vi "Parse Message Buffer.vi"(7 "flush buffer":bool, 8 "error in":errorcluster, 11 "string in":string) -> (0 "error out":errorcluster, 1 "valid":bool, 3 "message":T1)   [LabVIEW 2017, in "Lock-In Amplifier Example Shared.lvlib"]
uses:
  Lock-In Amplifier Example Shared.lvlib
  message.ctl
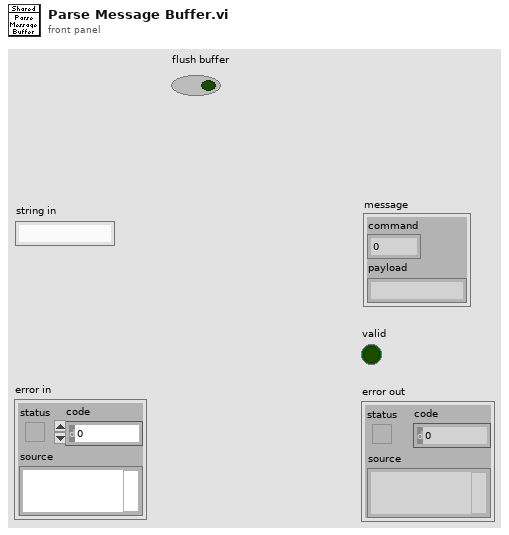
[diagram p1: front panel]
types:
  T1 = typedef "Lock-In Amplifier Example Shared.lvlib/message.ctl" = cluster{"command":u32, "payload":string}
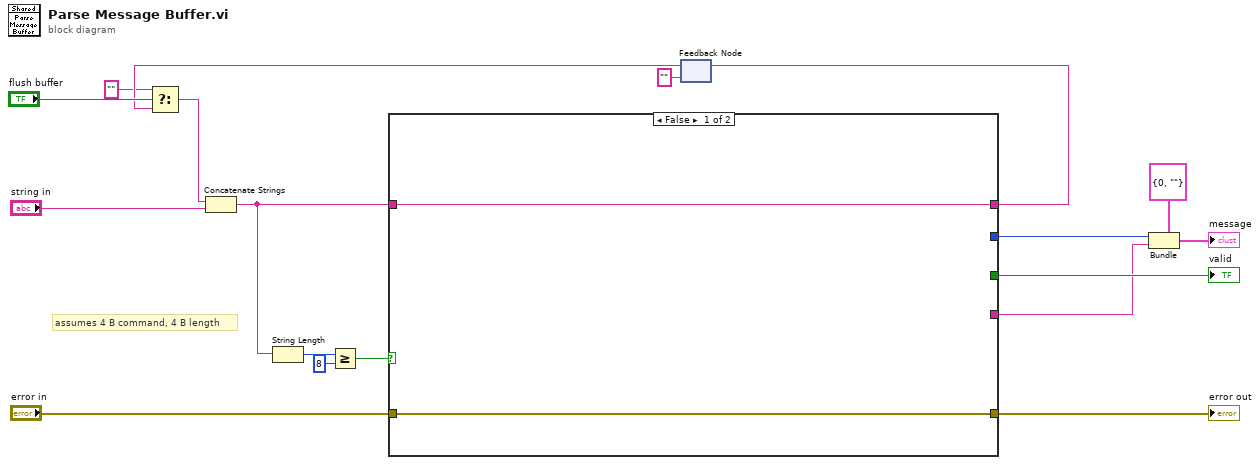
[diagram p0: block diagram]
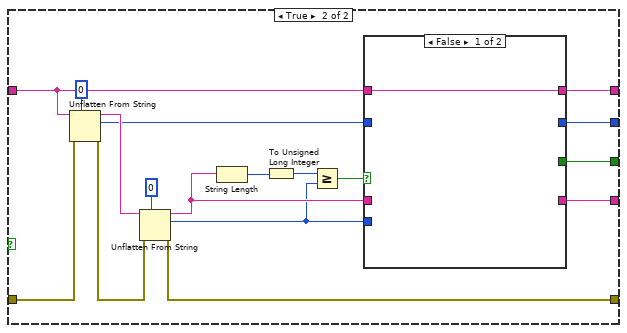
[diagram p2: hidden frame]
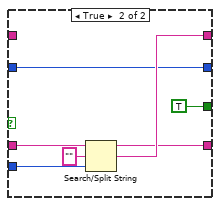
[diagram p3: hidden frame]
diagram:
  # "assumes 4 B command, 4 B length"
  n1 = feedback #1("") -> (w4:string)
  n2 = Select(t="", s="flush buffer", f=w4) -> (s? t:f=w2:string)
  n3 = Concatenate Strings(w2, "string in") -> (w13:string)
  n4 = String Length(string=w13) -> (length=w15:i32)
  n5 = Greater Or Equal?(x=w15, y=8) -> (x >= y?=w17:bool)
  n6 = case shown="False" w17 {
    tunnel: w13 -> [w20 w31]
    tunnel: [_ w30] -> w14
    tunnel: "error in" -> [w19 w29]
    tunnel: [w19 w27] -> w11
    tunnel: [w20 w24] -> w6
    tunnel: [_ w23] -> w9
    tunnel: [_ w21] -> w10
    frame False {
    }
    frame True {
      n7 = Unflatten From String(type=u32 0 ("offset (0)"), binary string=w31, error in (no error)=w29) -> (rest of the binary string=w36:string, value=w22:u32, error out=w28:errorcluster)  [unwired: 2 in]
      n8 = Unflatten From String(type=u32 0 ("offset (0)"), binary string=w36, error in (no error)=w28) -> (rest of the binary string=w26:string, value=w25:u32, error out=w27:errorcluster)  [unwired: 2 in]
      n9 = String Length(string=w26) -> (length=w34:i32)
      n10 = To Unsigned Long Integer(number=w34) -> (unsigned 32bit integer=w33:u32)
      n11 = Greater Or Equal?(x=w33, y=w25) -> (x >= y?=w32:bool)
      n12 = case shown="False" w32 {
        tunnel: w31 -> [w38 _]
        tunnel: [w38 w42] -> w24
        tunnel: [_ TRUE] -> w30
        tunnel: w26 -> [_ w45]
        tunnel: w25 -> [_ w44]
        tunnel: [_ w41] -> w23
        tunnel: w22 -> [_ w39]
        tunnel: [_ w39] -> w21
        frame False {
        }
        frame True {
          n13 = Search/Split String(string=w45, search string/char (-)="", offset (0)=w44) -> (substring before match=w41:string, match + rest of string=w42:string)  [unwired: 1 out]
        }
      }
    }
  }
  "error out" <- w11
  "valid" <- w14
  n14 = feedback-in #1(w6) -> ()
  n15 = Bundle(cluster=T1 {"command"=0, "payload"=""} ("message"), "command"=w10, "payload"=w9) -> (→"message":T1)
